vi "FPGA Read Control Scalar Address by Index.vi"(8 "error in (no error)":errorcluster, 9 "index":i32, 10 "Data Type":T1, 11 "FPGA Interface Base in":refnum<class "FPGA Interface Base.lvclass">) -> (0 "error out":errorcluster, 1 "Found?":bool, 2 "Address":u32, 3 "FPGA Interface Base out":refnum<class "FPGA Interface Base.lvclass">)   [LabVIEW 2010, in "FPGA Interface Base.lvclass"]
uses:
  <userlib>/_FPGA Interface Advanced Tools/FPGA Interface Base/FPGA Interface Base.lvclass
  <vilib>/rvi/DataTransferAndStorage/Container/Common/niFpgaDataTypeControl.ctl
  <userlib>/_FPGA Interface Advanced Tools/FPGA Interface Base/FPGA Interface Base.lvclass/FPGA Interface Base.ctl
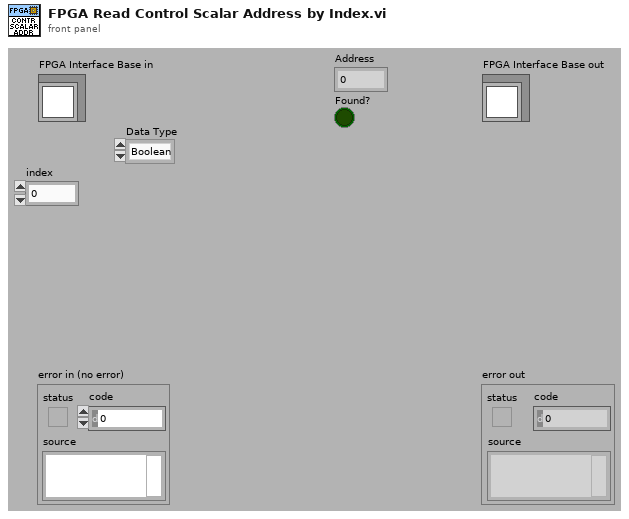
[diagram p1: front panel]
types:
  T1 = typedef "niFpgaDataTypeControl.ctl" = enum32{"Boolean", "I8", "I16", "I32", "I64", "U8", "U16", "U32", "U64", "FXP", "CustomControl"}
  T2 = typedef "FPGA Interface Base.lvclass/FPGA Session.ctl" = refnum<data-value>
  T3 = typedef "FPGA Interface Base.lvclass/FPGA Session Data.ctl" = cluster{"Session Out":u32, "Indicator Scalars":T4, "Indicator Arrays":T6, "Control Scalars":T4, "Control Arrays":T6, "TargetToHost FIFO Channels":T8, "HostToTarget FIFO Channels":T8, "All FIFOs":T9[], "IRQ Context Queue":refnum<queue>}
  T4 = typedef "FPGA Bitfile Utility.lvlib/Scalar Register Set.ctl" = cluster{"Boolean":T5[], "I8":T5[], "I16":T5[], "I32":T5[], "I64":T5[], "U8":T5[], "U16":T5[], "U32":T5[], "U64":T5[]}
  T5 = typedef "FPGA Bitfile Utility.lvlib/Scalar Register.ctl" = cluster{"Address":u32, "Name":string}
  T6 = typedef "FPGA Bitfile Utility.lvlib/Array Register Set.ctl" = cluster{"Boolean":T7[], "I8":T7[], "I16":T7[], "I32":T7[], "I64":T7[], "U8":T7[], "U16":T7[], "U32":T7[], "U64":T7[]}
  T7 = typedef "FPGA Bitfile Utility.lvlib/Array Register.ctl" = cluster{"Address":u32, "Num Elements":u32, "Name":string}
  T8 = typedef "FPGA Bitfile Utility.lvlib/FIFO Channel Set.ctl" = cluster{"Boolean":T9[], "I8":T9[], "I16":T9[], "I32":T9[], "I64":T9[], "U8":T9[], "U16":T9[], "U32":T9[], "U64":T9[]}
  T9 = typedef "FPGA Bitfile Utility.lvlib/FIFO Channel.ctl" = cluster{"Physical Channel":u32, "Name":string}
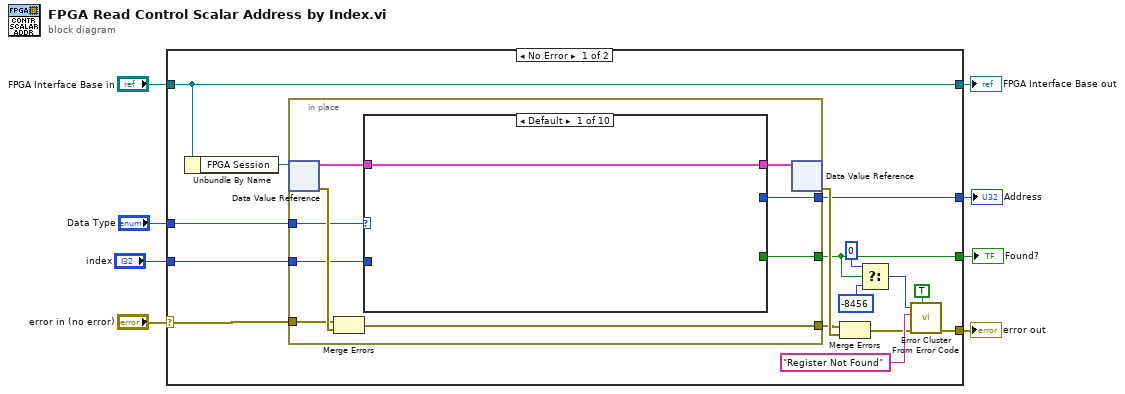
[diagram p0: block diagram]
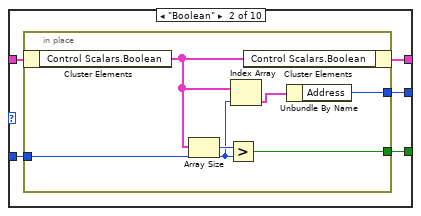
[diagram p2: hidden frame]
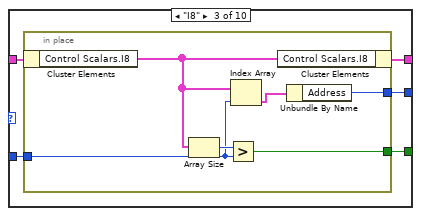
[diagram p3: hidden frame]
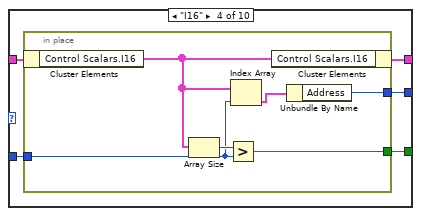
[diagram p4: hidden frame]
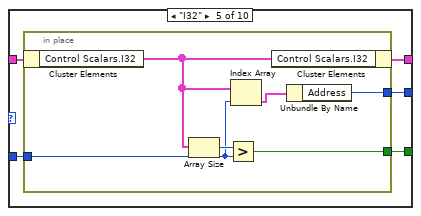
[diagram p5: hidden frame]
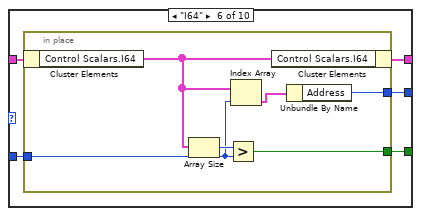
[diagram p6: hidden frame]
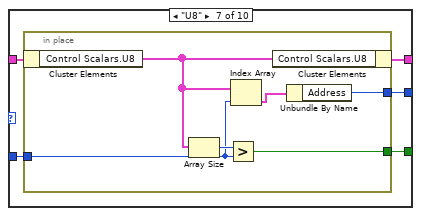
[diagram p7: hidden frame]
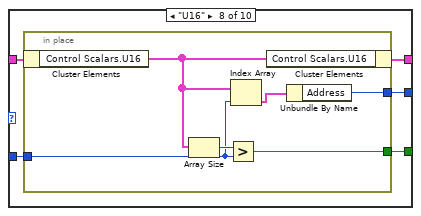
[diagram p8: hidden frame]
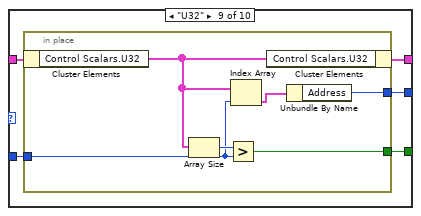
[diagram p9: hidden frame]
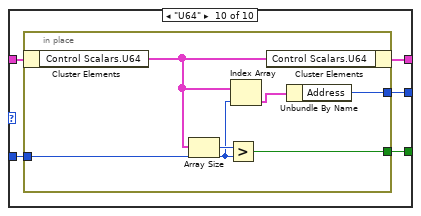
[diagram p10: hidden frame]
diagram:
  n1 = case shown="No Error" "error in (no error)" {
    selector: "error in (no error)" -> [w19 w134]
    tunnel: [w11 w134] -> w7
    tunnel: [w24 w135] -> w5
    tunnel: "FPGA Interface Base in" -> [w24 w135]
    tunnel: [w20 _] -> w4
    tunnel: [w9 _] -> w3
    tunnel: "Data Type" -> [w18 _]
    tunnel: "index" -> [w17 _]
    frame No Error {
      n2 = Unbundle By Name(w24) -> ("FPGA Session"=w21:T2)
      n3 = in-place {
        in-place-border: [w27] -> w20
        in-place-border: [w25] -> w9
        in-place-border: [w32] -> w22
        in-place-border: w19 -> [w31]
        in-place-border: w18 -> [w28]
        in-place-border: w17 -> [w29]
        n4 = in-place-dvr #1(w21) -> (w30:T3, w33:errorcluster)
        n5 = Merge Errors(w31, w33) -> (w32:errorcluster)
        n6 = case shown="Default" w28 {
          tunnel: w30 -> [w34 w39 w50 w61 w72 w83 w94 w105 w116 w127]
          tunnel: [w34 w38 w49 w60 w71 w82 w93 w104 w115 w126] -> w26
          tunnel: [_ w37 w48 w59 w70 w81 w92 w103 w114 w125] -> w27
          tunnel: [_ w36 w47 w58 w69 w80 w91 w102 w113 w124] -> w25
          tunnel: w29 -> [_ w35 w46 w57 w68 w79 w90 w101 w112 w123]
          frame Default {
          }
          frame "Boolean" {
            n7 = in-place {
              in-place-border: [w45] -> w37
              in-place-border: [w43] -> w36
              in-place-border: w35 -> [w40]
              n8 = in-place-cluster #2(w39) -> ("Control Scalars.Boolean"=w42:T5[])
              n9 = Array Size(array=w42) -> (size(s)=w44:i32)
              n10 = Greater?(x=w44, y=w40) -> (0:w43:bool)
              n11 = Index Array(array=w42, index=w40) -> (element=w41:T5)
              n12 = in-place-cluster #2("Control Scalars.Boolean"=w42) -> (w38:T3)
              n13 = Unbundle By Name(w41) -> ("Address"=w45:u32)
            }
          }
          frame "I8" {
            n14 = in-place {
              in-place-border: [w56] -> w48
              in-place-border: [w54] -> w47
              in-place-border: w46 -> [w51]
              n15 = in-place-cluster #3(w50) -> ("Control Scalars.I8"=w53:T5[])
              n16 = Array Size(array=w53) -> (size(s)=w55:i32)
              n17 = Greater?(x=w55, y=w51) -> (0:w54:bool)
              n18 = Index Array(array=w53, index=w51) -> (element=w52:T5)
              n19 = in-place-cluster #3("Control Scalars.I8"=w53) -> (w49:T3)
              n20 = Unbundle By Name(w52) -> ("Address"=w56:u32)
            }
          }
          frame "I16" {
            n21 = in-place {
              in-place-border: [w67] -> w59
              in-place-border: [w65] -> w58
              in-place-border: w57 -> [w62]
              n22 = in-place-cluster #4(w61) -> ("Control Scalars.I16"=w64:T5[])
              n23 = Array Size(array=w64) -> (size(s)=w66:i32)
              n24 = Greater?(x=w66, y=w62) -> (0:w65:bool)
              n25 = Index Array(array=w64, index=w62) -> (element=w63:T5)
              n26 = in-place-cluster #4("Control Scalars.I16"=w64) -> (w60:T3)
              n27 = Unbundle By Name(w63) -> ("Address"=w67:u32)
            }
          }
          frame "I32" {
            n28 = in-place {
              in-place-border: [w78] -> w70
              in-place-border: [w76] -> w69
              in-place-border: w68 -> [w73]
              n29 = in-place-cluster #5(w72) -> ("Control Scalars.I32"=w75:T5[])
              n30 = Array Size(array=w75) -> (size(s)=w77:i32)
              n31 = Greater?(x=w77, y=w73) -> (0:w76:bool)
              n32 = Index Array(array=w75, index=w73) -> (element=w74:T5)
              n33 = in-place-cluster #5("Control Scalars.I32"=w75) -> (w71:T3)
              n34 = Unbundle By Name(w74) -> ("Address"=w78:u32)
            }
          }
          frame "I64" {
            n35 = in-place {
              in-place-border: [w89] -> w81
              in-place-border: [w87] -> w80
              in-place-border: w79 -> [w84]
              n36 = in-place-cluster #6(w83) -> ("Control Scalars.I64"=w86:T5[])
              n37 = Array Size(array=w86) -> (size(s)=w88:i32)
              n38 = Greater?(x=w88, y=w84) -> (0:w87:bool)
              n39 = Index Array(array=w86, index=w84) -> (element=w85:T5)
              n40 = in-place-cluster #6("Control Scalars.I64"=w86) -> (w82:T3)
              n41 = Unbundle By Name(w85) -> ("Address"=w89:u32)
            }
          }
          frame "U8" {
            n42 = in-place {
              in-place-border: [w100] -> w92
              in-place-border: [w98] -> w91
              in-place-border: w90 -> [w95]
              n43 = in-place-cluster #7(w94) -> ("Control Scalars.U8"=w97:T5[])
              n44 = Array Size(array=w97) -> (size(s)=w99:i32)
              n45 = Greater?(x=w99, y=w95) -> (0:w98:bool)
              n46 = Index Array(array=w97, index=w95) -> (element=w96:T5)
              n47 = in-place-cluster #7("Control Scalars.U8"=w97) -> (w93:T3)
              n48 = Unbundle By Name(w96) -> ("Address"=w100:u32)
            }
          }
          frame "U16" {
            n49 = in-place {
              in-place-border: [w111] -> w103
              in-place-border: [w109] -> w102
              in-place-border: w101 -> [w106]
              n50 = in-place-cluster #8(w105) -> ("Control Scalars.U16"=w108:T5[])
              n51 = Array Size(array=w108) -> (size(s)=w110:i32)
              n52 = Greater?(x=w110, y=w106) -> (0:w109:bool)
              n53 = Index Array(array=w108, index=w106) -> (element=w107:T5)
              n54 = in-place-cluster #8("Control Scalars.U16"=w108) -> (w104:T3)
              n55 = Unbundle By Name(w107) -> ("Address"=w111:u32)
            }
          }
          frame "U32" {
            n56 = in-place {
              in-place-border: [w122] -> w114
              in-place-border: [w120] -> w113
              in-place-border: w112 -> [w117]
              n57 = in-place-cluster #9(w116) -> ("Control Scalars.U32"=w119:T5[])
              n58 = Array Size(array=w119) -> (size(s)=w121:i32)
              n59 = Greater?(x=w121, y=w117) -> (0:w120:bool)
              n60 = Index Array(array=w119, index=w117) -> (element=w118:T5)
              n61 = in-place-cluster #9("Control Scalars.U32"=w119) -> (w115:T3)
              n62 = Unbundle By Name(w118) -> ("Address"=w122:u32)
            }
          }
          frame "U64" {
            n63 = in-place {
              in-place-border: [w133] -> w125
              in-place-border: [w131] -> w124
              in-place-border: w123 -> [w128]
              n64 = in-place-cluster #10(w127) -> ("Control Scalars.U64"=w130:T5[])
              n65 = Array Size(array=w130) -> (size(s)=w132:i32)
              n66 = Greater?(x=w132, y=w128) -> (0:w131:bool)
              n67 = Index Array(array=w130, index=w128) -> (element=w129:T5)
              n68 = in-place-cluster #10("Control Scalars.U64"=w130) -> (w126:T3)
              n69 = Unbundle By Name(w129) -> ("Address"=w133:u32)
            }
          }
        }
        n70 = in-place-dvr #1(w26) -> (w23:errorcluster)  [unwired: 1 out]
      }
      n71 = Merge Errors(w22, w23) -> (w10:errorcluster)
      n72 = Select(t=0, s=w9, f=-8456 ("error code (0)")) -> (s? t:f=w15:i32)
      n73 = call <vilib>:"Error Cluster From Error Code.vi"("show call chain? (False)"=TRUE, "error in (no error)"=w10, "error message (\"\")"="Register Not Found" ("string"), "error code (0)"=w15) -> ("error out"=w11:errorcluster)  [unwired: 5 in]
    }
    frame Error {
    }
  }
  "error out" <- w7
  "FPGA Interface Base out" <- w5
  "Address" <- w4
  "Found?" <- w3
